vi "Read Temp.vi"(8 "error in (no error)":errorcluster, 11 "Bronkhorst Settings in":T1) -> (0 "error out":errorcluster, 1 "Connection Error":bool, 2 "Temp (C)":sgl, 3 "Bronkhorst Settings out":T1)   [LabVIEW 2018]
uses:
  Bronkhorst M13 Flow Meter/Settings Cluster.ctl
  <vilib>/regexp/Match Regular Expression.xnode
  <vilib>/ptbypt/NI_PtbyPt.lvlib
  Bronkhorst M13 Flow Meter/Bronkhorst M13 Flow Meter.lvlib
panel:
  out "read buffer":string
  out "whole match":string
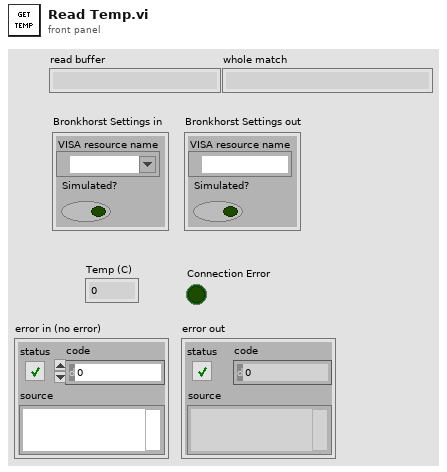
[diagram p1: front panel]
types:
  T1 = typedef "Bronkhorst M13 Flow Meter.lvlib/Settings Cluster.ctl" = cluster{"VISA resource name":refnum<visa-resource-name>, "Simulated?":bool}
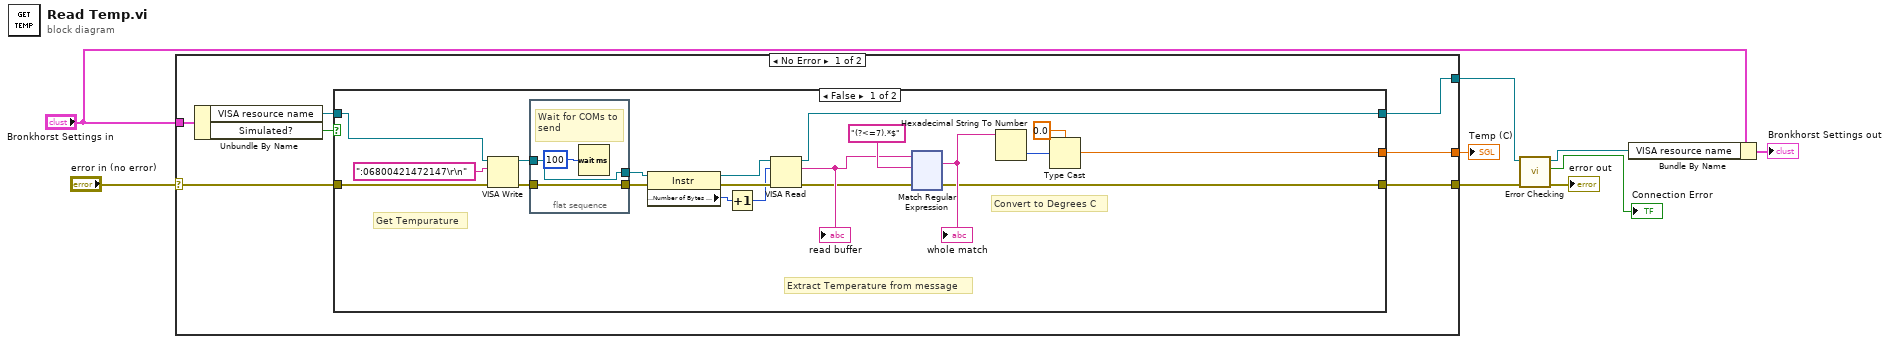
[diagram p0: block diagram]
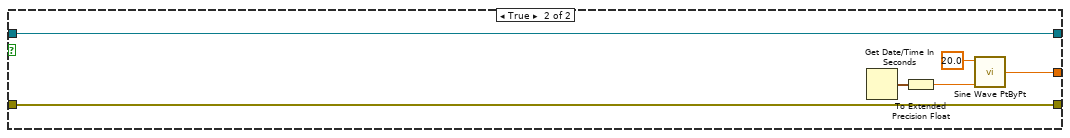
[diagram p2: hidden frame]
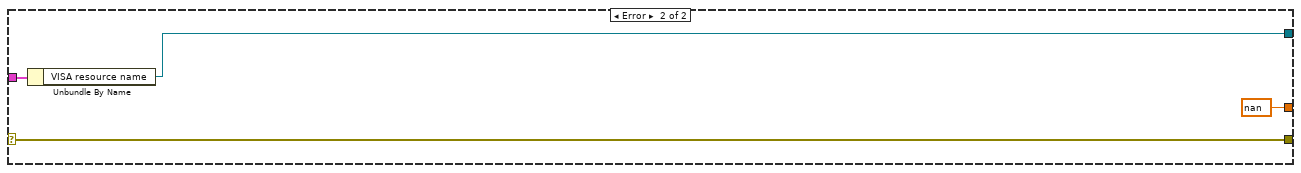
[diagram p3: hidden frame]
diagram:
  n1 = case shown="No Error" "error in (no error)" {
    selector: "error in (no error)" -> [w15 w163]
    tunnel: [w14 w163] -> w4
    tunnel: "Bronkhorst Settings in" -> [w13 w162]
    tunnel: [w11 w161] -> w6
    tunnel: [w10 nan ("sine wave")] -> w1
    frame No Error {
      n2 = Unbundle By Name(w13) -> ("VISA resource name"=w12:refnum<visa-resource-name>, "Simulated?"=w16:bool)
      n3 = case shown="False" w16 {
        tunnel: [w17 w159] -> w14
        tunnel: w15 -> [w28 w159]
        tunnel: [w25 w155] -> w11
        tunnel: w12 -> [w29 w155]
        tunnel: [w22 w154] -> w10
        frame False {
          # "Extract Temperature from message"
          # "Get Tempurature"
          # "Convert to Degrees C"
          n4 = VISA Write(VISA resource name=w29, write buffer=":06800421472147\r\n" ("Command"), error in (no error)=w28) -> (VISA resource name out=w33:refnum<visa-resource-name>, error out=w31:errorcluster)  [unwired: 1 out]
          n5 = flat-sequence {
            tunnel: [w153] -> w32
            tunnel: w33 -> [w153]
            tunnel: [w152] -> w30
            tunnel: w31 -> [w152]
            frame #0 {
              # "Wait for COMs to send"
              n6 = Wait (ms)(milliseconds to wait=u32 100) -> ()  [unwired: 1 out]
            }
          }
          n7 = property class="Instr"(reference=w32, error in=w30) -> (reference out=w35:refnum<visa-resource-name>, error out=w34:errorcluster, "Serial Settings:Number of Bytes at Serial Port"=w27:u32)
          n8 = Increment(x=w27) -> (x+1=w26:u32)
          n9 = VISA Read(VISA resource name=w35, byte count=w26, error in (no error)=w34) -> (VISA resource name out=w25:refnum<visa-resource-name>, read buffer=w20:string, error out=w18:errorcluster)  [unwired: 1 out]
          "read buffer" <- w20
          n10 = xnode "Match Regular Expression"("input string"=w20, "regular expression"="(?<=7).*$" ("Regular Expression for Extracting Weight"), "error in"=w18) -> ("whole match"=w19:string, "error out"=w17:errorcluster)  [unwired: 3 in, 3 out]
          "whole match" <- w19
          n11 = Hexadecimal String To Number(string=w19) -> (number=w23:u32)  [unwired: 2 in, 1 out]
          n12 = Type Cast(type=sgl 0.0, x=w23) -> (*(type *) &x=w22:sgl)
        }
        frame True {
          n13 = Get Date/Time In Seconds() -> (seconds since 1Jan1904=w158:timestamp)
          n14 = To Extended Precision Float(1:w158) -> (0:w157:ext)
          n15 = call <vilib>:"Sine Wave PtByPt.vi"("time"=w157, "amplitude"=20.0) -> ("sine wave"=w154:dbl)  [unwired: 2 in]
        }
      }
    }
    frame Error {
      n16 = Unbundle By Name(w162) -> ("VISA resource name"=w161:refnum<visa-resource-name>)
    }
  }
  "Temp (C)" <- w1
  n17 = call "Error Checking.vi"("error in (no error)"=w4, "VISA resource name"=w6) -> ("error out"=→"error out":errorcluster, "Connection Error"=→"Connection Error":bool, "VISA resource name"=w5:refnum<visa-resource-name>)  [unwired: 7 in]
  n18 = Bundle By Name(cluster="Bronkhorst Settings in", "VISA resource name"=w5) -> (→"Bronkhorst Settings out":T1)
